vi "EOL Test.vi"() -> ()   [LabVIEW 2017]
panel:
  out "offset (in bytes)":i64=1501
  out "file out":i32=1501
  out "file in":i32=1501
  in  "String":string="HEADER,TR Address, RF Direction,Select Command, Phase Shift (deg), Attenuation (dB), Temperature (C),Date,Time,\n,0,Tx,Vertical,0.000,0.000,23.5,2015/07/23,23:59:02\r\nFreq(Hz),S11(DB),S11(DEG),S12(DB),S12(DEG),S21(DB),S21(DEG),S22(DB),S22(DEG)\r\n5000000000,-42.771954,152.22778,0.082412034,-0.52403092,0.030667592,0.65514064,-48.369854,61.337074\r\n5005000000,-46.862316,169.26343,0.081046775,-0.41602013,0.033997945,0.62726825,-46.838844,49.065746\r\n5010000000,-44.007118,171.36211,0.08570607,-0.50450921,0.027771581,0.60231954,-48.501251,34.107002\r\n5015000000,-44.942177,170.8213,0.076357558,-0.55446047,0.029190876,0.58199483,-46.526299,31.423214\r\n5020000000,-46.815594,165.79419,0.080755487,-0.48572463,0.025612796,0.63927662,-48.603924,34.328793\r\n5025000000,-43.415237,160.28862,0.083058313,-0.45693678,0.029641846,0.59327209,-50.967751,62.951927\r\n5030000000,-42.987732,167.38646,0.084096409,-0.61792517,0.022725577,0.60476542,-46.619244,32.048206\r\n5035000000,-42.430008,142.06786,0.075368881,-0.47846141,0.03584785,0.64242035,-47.592979,62.97485\r\n5040000000,-42.209286,178.73824,0.06679257,-0.56306696,0.026645718,0.66881263,-49.586189,41.288471\r\n5045000000,-43.148418,159.36703,0.07832209,-0.50556082,0.019004442,0.63425356,-48.029884,51.484097\r\n5050000000,-42.476814,150.24446,0.075575255,-0.53875768,0.031528965,0.60036933,-47.000137,60.907242\r\n5055000000,-44.583641,144.83051,0.088081352,-0.4841038,0.018026941,0.60976517,-54.021416,68.02684\r\n5060000000,-39.945629,143.52361,0.078626417,-0.5605384"
  out "text":string="HEADER,TR Address, RF Direction,Select Command, Phase Shift (deg), Attenuation (dB), Temperature (C),Date,Time,\n,0,Tx,Vertical,0.000,0.000,23.5,2015/07/23,23:59:02\r\nFreq(Hz),S11(DB),S11(DEG),S12(DB),S12(DEG),S21(DB),S21(DEG),S22(DB),S22(DEG)\r\n5000000000,-42.771954,152.22778,0.082412034,-0.52403092,0.030667592,0.65514064,-48.369854,61.337074\r\n5005000000,-46.862316,169.26343,0.081046775,-0.41602013,0.033997945,0.62726825,-46.838844,49.065746\r\n5010000000,-44.007118,171.36211,0.08570607,-0.50450921,0.027771581,0.60231954,-48.501251,34.107002\r\n5015000000,-44.942177,170.8213,0.076357558,-0.55446047,0.029190876,0.58199483,-46.526299,31.423214\r\n5020000000,-46.815594,165.79419,0.080755487,-0.48572463,0.025612796,0.63927662,-48.603924,34.328793\r\n5025000000,-43.415237,160.28862,0.083058313,-0.45693678,0.029641846,0.59327209,-50.967751,62.951927\r\n5030000000,-42.987732,167.38646,0.084096409,-0.61792517,0.022725577,0.60476542,-46.619244,32.048206\r\n5035000000,-42.430008,142.06786,0.075368881,-0.47846141,0.03584785,0.64242035,-47.592979,62.97485\r\n5040000000,-42.209286,178.73824,0.06679257,-0.56306696,0.026645718,0.66881263,-49.586189,41.288471\r\n5045000000,-43.148418,159.36703,0.07832209,-0.50556082,0.019004442,0.63425356,-48.029884,51.484097\r\n5050000000,-42.476814,150.24446,0.075575255,-0.53875768,0.031528965,0.60036933,-47.000137,60.907242\r\n5055000000,-44.583641,144.83051,0.088081352,-0.4841038,0.018026941,0.60976517,-54.021416,68.02684\r\n5060000000,-39.945629,143.52361,0.078626417,-0.5605384"
  out "error out":errorcluster
  in  "file (use dialog)":path=path "C:/Users/Chris Clark/Documents/dummy2.txt"
  # "Both EOL       source \\r\\n converts to \\n, read string < read file offset\nBoth not EOL  source \\r\\n and \\n converts to same in read file\n\nWrite EOL, Read not   \\n is converted to \\r\\n\n                                       write len = 1501     read len = 1502\n Write not, Read EOL   source \\r\\n converts to \\n\n                                         write len = 1501     read len = 1487 read file offset = 1501"
  # "removinf EOL from both ascii write and read = what goes in = what comes out = file positions"
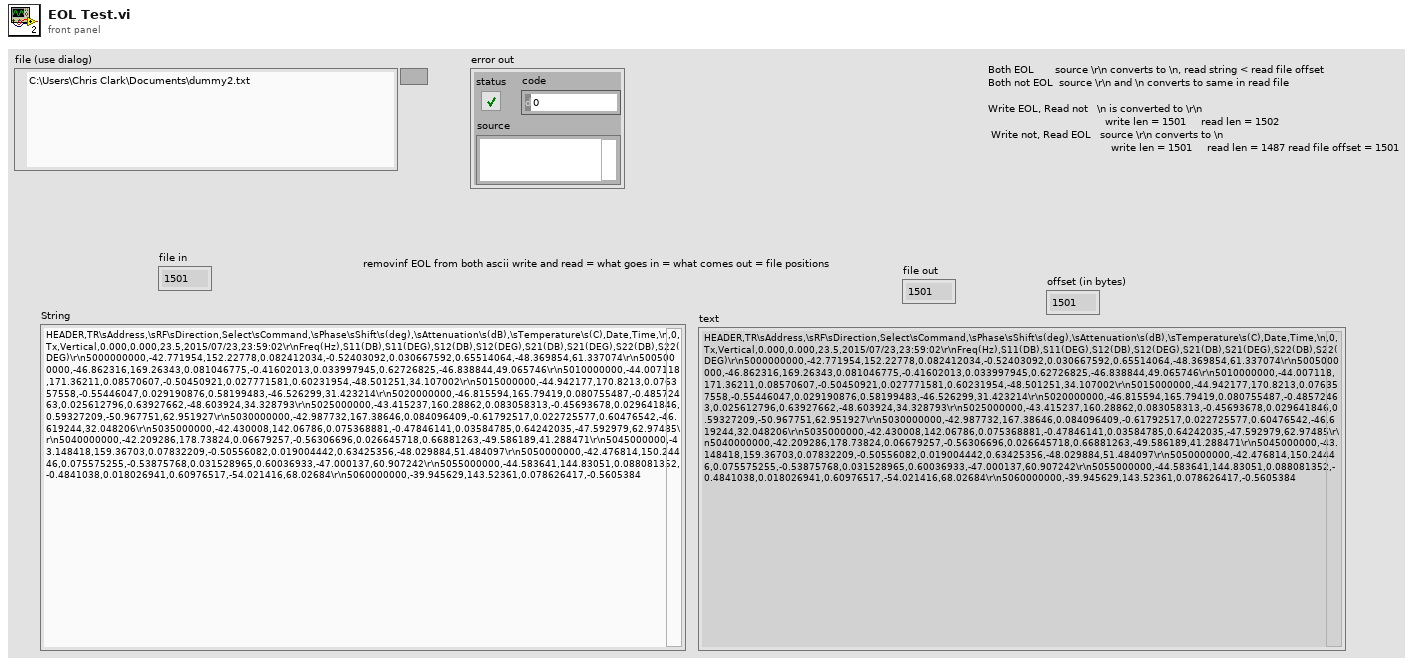
[diagram p1: front panel]
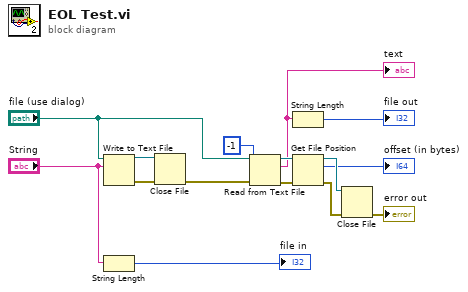
[diagram p0: block diagram]
diagram:
  n1 = Write to Text File(file (use dialog)="file (use dialog)", text="String") -> (refnum out=w3:refnum<file>, error out=w4:errorcluster)  [unwired: 2 in, 1 out]
  n2 = String Length(string="String") -> (length=→"file in":i32)
  n3 = Close File(refnum=w3, error in=w4) -> (error out=w2:errorcluster)  [unwired: 1 out]
  n4 = Read from Text File(file (use dialog)="file (use dialog)", count=-1, error in=w2) -> (refnum out=w13:refnum<file>, text=w7:string, error out=w14:errorcluster)  [unwired: 1 in, 1 out]
  "text" <- w7
  n5 = String Length(string=w7) -> (length=→"file out":i32)
  n6 = Get File Position(4:w14, 7:w13) -> (0:w12:errorcluster, 2:→"offset (in bytes)":i64, 3:w11:refnum<file>)
  n7 = Close File(refnum=w11, error in=w12) -> (error out=→"error out":errorcluster)  [unwired: 1 out]
